vi "read-json-testing.vi"() -> ()   [LabVIEW 2019]
panel:
  out "value":T1(array[cluster])
  in  "trajectory":T1(array[cluster])
  in  "enable LabVIEW extensions? (T)":bool=TRUE
  in  "strict validation? (F)":bool
  in  "default null elements? (F)":bool=TRUE
  out "error out":errorcluster
  in  "path":string[](array[string])
  in  "json source":string="[\n    {\n        \"timestamp\": 0,\n        \"x\": 5.982723236083984,\n        \"y\": 3.8337526321411137,\n        \"heading\": -0.02726589531195272,\n        \"velocityX\": 0,\n        \"velocityY\": 9.683808101189284e-35,\n        \"angularVelocity\": 0\n    },\n    {\n        \"timestamp\": 0.03810324695055001,\n        \"x\": 5.98684701120518,\n        \"y\": 3.836695144747058,\n        \"heading\": -0.02635908015583591,\n        \"velocityX\": 0.10822634424167109,\n        \"velocityY\": 0.07722472076364896,\n        \"angularVelocity\": 0.023798894548105808\n    },\n    {\n        \"timestamp\": 0.07620649390110001,\n        \"x\": 5.9951102276307955,\n        \"y\": 3.842555990890375,\n        \"heading\": -0.02450943734161065,\n        \"velocityX\": 0.21686383935573297,\n        \"velocityY\": 0.15381487438388347,\n        \"angularVelocity\": 0.048542918576604074\n    },\n    {\n        \"timestamp\": 0.11430974085165002,\n        \"x\": 6.007530540708913,\n        \"y\": 3.851307449548468,\n        \"heading\": -0.021675911820365212,\n        \"velocityX\": 0.3259646899445822,\n        \"velocityY\": 0.2296775041100852,\n        \"angularVelocity\": 0.07436441112018764\n    },\n    {\n        \"timestamp\": 0.15241298780220003,\n        \"x\": 6.024127990876516,\n        \"y\": 3.8629174242827835,\n        \"heading\": -0.017811264169326626,\n        \"velocityX\": 0.43559149143231607,\n        \"velocityY\": 0.3046977794145049,\n        \"angularVelocity\": 0.10142567787079011\n    },\n    {\n        \"timestamp\": 0.19051623475275004,\n        \"x\": 6.044925508435204,\n        \"y\": 3.8773483282979404,\n        \"heading\": -0.0128605531052204,\n        \"velocityX\": 0.5458200868203993,\n        \"velocityY\": 0.37873160872313927,\n        \"angularVelocity\": 0.12992885017200875\n    },\n    {\n        \"timestamp\": 0.22861948170330004,\n        \"x\": 6.0699495650843565,\n        \"y\": 3.894555559389049,\n        \"heading\": -0.006759072154586934,\n        \"velocityX\": 0.6567434182611646,\n        \"velocityY\": 0.45159487624347117,\n        \"angularVelocity\": 0.16013021038733294\n    },\n    {\n        \"timestamp\": 0.26672272865385005,\n        \"x\": 6.0992310251847055,\n        \"y\": 3.91448535931083,\n        \"heading\": 0.0005705329934009674,\n        \"velocityX\": 0.7684767688787957,\n        \"velocityY\": 0.5230472864332357,\n        \"angularVelocity\": 0.19236169446395399\n    },\n    {\n        \"timestamp\": 0.30482597560440006,\n        \"x\": 6.132806269868785,\n        \"y\": 3.9370717165814155,\n        \"heading\": 0.009222426006961602,\n        \"velocityX\": 0.8811649234946475,\n        \"velocityY\": 0.5927672594384606,\n        \"angularVelocity\": 0.2270644552887354\n    },\n    {\n        \"timestamp\": 0.34292922255495006,\n        \"x\": 6.170718689966367,\n        \"y\": 3.962231721071589,\n        \"heading\": 0.01931383560441445,\n        \"velocityX\": 0.9949918479857032,\n        \"velocityY\": 0.6603112990035996,\n        \"angularVelocity\": 0.2648438231667591\n    },\n    {\n        \"timestamp\": 0.38103246950550007,\n        \"x\": 6.213020653091169,\n        \"y\": 3.989858289069104,\n        \"heading\": 0.030994951202651673,\n        \"velocityX\": 1.1101931334015223,\n        \"velocityY\": 0.7250449819504136,\n        \"angularVelocity\": 0.3065648345768179\n    },\n    {\n        \"timestamp\": 0.4191357164560501,\n        \"x\": 6.259775973212591,\n        \"y\": 4.019808160211835,\n        \"heading\": 0.04446563724227389,\n        \"velocityX\": 1.2270691834242344,\n        \"velocityY\": 0.7860188708221707,\n        \"angularVelocity\": 0.3535311848122014\n    },\n    {\n        \"timestamp\": 0.4572389634066001,\n        \"x\": 6.311062435579481,\n        \"y\": 4.051880814371457,\n        \"heading\": 0.060006160684953305,\n        \"velocityX\": 1.3459866670536105,\n        \"velocityY\": 0.8417302126835429,\n        \"angularVelocity\": 0.40785299643479905\n    },\n    {\n        \"timestamp\": 0.4953422103571501,\n        \"x\": 6.366971668412108,\n        \"y\": 4.085778739706103,\n        \"heading\": 0.0780398678585479,\n        \"velocityX\": 1.4673088859116663,\n        \"velocityY\": 0.8896335102002109,\n        \"angularVelocity\": 0.47328531337489643\n    },\n    {\n        \"timestamp\": 0.5334454573077001,\n        \"x\": 6.42759324409593,\n        \"y\": 4.1210284288786045,\n        \"heading\": 0.09927318993914273,\n        \"velocityX\": 1.5909818856775562,\n        \"velocityY\": 0.9251098526654346,\n        \"angularVelocity\": 0.5572575509942492\n    },\n    {\n        \"timestamp\": 0.5715487042582501,\n        \"x\": 6.492929850638083,\n        \"y\": 4.156837507973627,\n        \"heading\": 0.12496268004834134,\n        \"velocityX\": 1.7147254307998017,\n        \"velocityY\": 0.9397907517301461,\n        \"angularVelocity\": 0.6742073750968268\n    },\n    {\n        \"timestamp\": 0.6096519512088001,\n        \"x\": 6.562698684949471,\n        \"y\": 4.191947985905663,\n        \"heading\": 0.1565497680971661,\n        \"velocityX\": 1.8310469551829356,\n        \"velocityY\": 0.9214563256930572,\n        \"angularVelocity\": 0.8289867813578368\n    },\n    {\n        \"timestamp\": 0.6477551981593501,\n        \"x\": 6.635139463079909,\n        \"y\": 4.223639351259096,\n        \"heading\": 0.19449877991768647,\n        \"velocityX\": 1.9011707381381133,\n        \"velocityY\": 0.8317234852599791,\n        \"angularVelocity\": 0.9959521788203487\n    },\n    {\n        \"timestamp\": 0.6858584451099001,\n        \"x\": 6.7081933797465005,\n        \"y\": 4.250935758839449,\n        \"heading\": 0.23877166971400077,\n        \"velocityX\": 1.917262241755836,\n        \"velocityY\": 0.7163800926409031,\n        \"angularVelocity\": 1.1619190840553386\n    },\n    {\n        \"timestamp\": 0.7239616920604501,\n        \"x\": 6.780136139474193,\n        \"y\": 4.273495418390116,\n        \"heading\": 0.28647328812510897,\n        \"velocityX\": 1.888100502853595,\n        \"velocityY\": 0.5920665915937995,\n        \"angularVelocity\": 1.2519042923826915\n    },\n    {\n        \"timestamp\": 0.7620649390110001,\n        \"x\": 6.850045632550813,\n        \"y\": 4.291512251071874,\n        \"heading\": 0.3365456853758495,\n        \"velocityX\": 1.8347384716936121,\n        \"velocityY\": 0.47284245106833517,\n        \"angularVelocity\": 1.3141241562884853\n    },\n    {\n        \"timestamp\": 0.8001681859615501,\n        \"x\": 6.9174385893155375,\n        \"y\": 4.305183550968592,\n        \"heading\": 0.3884190669725829,\n        \"velocityX\": 1.7686932783493219,\n        \"velocityY\": 0.35879619168575444,\n        \"angularVelocity\": 1.3613900585442669\n    },\n    {\n        \"timestamp\": 0.8382714329121002,\n        \"x\": 6.982024412284714,\n        \"y\": 4.314663617385671,\n        \"heading\": 0.44170912410253604,\n        \"velocityX\": 1.6950215044138437,\n        \"velocityY\": 0.24879943773254676,\n        \"angularVelocity\": 1.398569974866313\n    },\n    {\n        \"timestamp\": 0.8763746798626502,\n        \"x\": 7.043611527543253,\n        \"y\": 4.320071315528175,\n        \"heading\": 0.49614021122658447,\n        \"velocityX\": 1.616321972205263,\n        \"velocityY\": 0.14192223958037933,\n        \"angularVelocity\": 1.4285157166445919\n    },\n    {\n        \"timestamp\": 0.9144779268132002,\n        \"x\": 7.102065214635615,\n        \"y\": 4.32149953061112,\n        \"heading\": 0.5515071646371278,\n        \"velocityX\": 1.5340867713510038,\n        \"velocityY\": 0.037482765833582746,\n        \"angularVelocity\": 1.4530770430772049\n    },\n    {\n        \"timestamp\": 0.9525811737637502,\n        \"x\": 7.157286057818237,\n        \"y\": 4.319022257662232,\n        \"heading\": 0.6076525295540515,\n        \"velocityX\": 1.4492424557488948,\n        \"velocityY\": -0.06501474669864526,\n        \"angularVelocity\": 1.4735060502794106\n    },\n    {\n        \"timestamp\": 0.9906844207143002,\n        \"x\": 7.209197910760983,\n        \"y\": 4.312699565476428,\n        \"heading\": 0.664452255224938,\n        \"velocityX\": 1.362399719113554,\n        \"velocityY\": -0.1659357847904016,\n        \"angularVelocity\": 1.4906794096734857\n    },\n    {\n        \"timestamp\": 1.0287876676648502,\n        \"x\": 7.2577407022992615,\n        \"y\": 4.302581057423054,\n        \"heading\": 0.7218063948940598,\n        \"velocityX\": 1.2739804458469486,\n        \"velocityY\": -0.2655550081205459,\n        \"angularVelocity\": 1.5052297181801246\n    },\n    {\n        \"timestamp\": 1.0668909146154002,\n        \"x\": 7.3028658963835795,\n        \"y\": 4.288708316667104,\n        \"heading\": 0.779632866785423,\n        \"velocityX\": 1.184287369075913,\n        \"velocityY\": -0.3640829028022947,\n        \"angularVelocity\": 1.51762583294836\n    },\n    {\n        \"timestamp\": 1.1049941615659502,\n        \"x\": 7.344533497015384,\n        \"y\": 4.271116666027759,\n        \"heading\": 0.8378631451292572,\n        \"velocityX\": 1.0935446180184787,\n        \"velocityY\": -0.4616837683721217,\n        \"angularVelocity\": 1.5282235243470785\n    },\n    {\n        \"timestamp\": 1.1430974085165002,\n        \"x\": 7.3827099980564315,\n        \"y\": 4.249836459267662,\n        \"heading\": 0.8964392046934532,\n        \"velocityX\": 1.0019225157003373,\n        \"velocityY\": -0.5584880151477051,\n        \"angularVelocity\": 1.537298373553775\n    },\n    {\n        \"timestamp\": 1.1812006554670502,\n        \"x\": 7.417366935383198,\n        \"y\": 4.22489404631923,\n        \"heading\": 0.9553113025588683,\n        \"velocityX\": 0.9095533871888511,\n        \"velocityY\": -0.6546007215816033,\n        \"angularVelocity\": 1.5450677455866486\n    },\n    {\n        \"timestamp\": 1.2193039024176002,\n        \"x\": 7.448479836830729,\n        \"y\": 4.1963125073290035,\n        \"heading\": 1.014436333735295,\n        \"velocityX\": 0.816541999371032,\n        \"velocityY\": -0.7501077015120999,\n        \"angularVelocity\": 1.551705849455849\n    },\n    {\n        \"timestamp\": 1.2574071493681502,\n        \"x\": 7.4760274429392135,\n        \"y\": 4.164112219770215,\n        \"heading\": 1.0737765893932227,\n        \"velocityX\": 0.7229726680310206,\n        \"velocityY\": -0.8450798852018467,\n        \"angularVelocity\": 1.5573543046066753\n    },\n    {\n        \"timestamp\": 1.2955103963187002,\n        \"x\": 7.49999111698165,\n        \"y\": 4.12831130292246,\n        \"heading\": 1.1332988035654967,\n        \"velocityX\": 0.628914225434282,\n        \"velocityY\": -0.9395765377742389,\n        \"angularVelocity\": 1.5621297116627306\n    },\n    {\n        \"timestamp\": 1.3336136432692502,\n        \"x\": 7.520354390382808,\n        \"y\": 4.08892597080947,\n        \"heading\": 1.1929734104345324,\n        \"velocityX\": 0.5344235736021341,\n        \"velocityY\": -1.0336476616835946,\n        \"angularVelocity\": 1.566129179134875\n    },\n    {\n        \"timestamp\": 1.3717168902198003,\n        \"x\": 7.537102606975847,\n        \"y\": 4.045970815789375,\n        \"heading\": 1.252773957923772,\n        \"velocityX\": 0.43954827825499565,\n        \"velocityY\": -1.1273358167045713,\n        \"angularVelocity\": 1.5694344255451789\n    },\n    {\n        \"timestamp\": 1.4098201371703503,\n        \"x\": 7.550222640729637,\n        \"y\": 3.999459038895289,\n        \"heading\": 1.312676639030204,\n        \"velocityX\": 0.3443284970127743,\n        \"velocityY\": -1.2206775174422342,\n        \"angularVelocity\": 1.5721148694801685\n    },\n    {\n        \"timestamp\": 1.4479233841209003,\n        \"x\": 7.5597026689810605,\n        \"y\": 3.9494026387764034,\n        \"heading\": 1.3726599130276154,\n        \"velocityX\": 0.24879843609460844,\n        \"velocityY\": -1.313704319840455,\n        \"angularVelocity\": 1.574229988201789\n    },\n    {\n        \"timestamp\": 1.4860266310714503,\n        \"x\": 7.56553198821413,\n        \"y\": 3.8958125680834574,\n        \"heading\": 1.4327041960899756,\n        \"velocityX\": 0.15298746693777887,\n        \"velocityY\": -1.4064436755874,\n        \"angularVelocity\": 1.5758311395427256\n    },\n    {\n        \"timestamp\": 1.5241298780220003,\n        \"x\": 7.5677008628845215,\n        \"y\": 3.8386988639831543,\n        \"heading\": 1.492791606127603,\n        \"velocityX\": 0.05692099345774061,\n        \"velocityY\": -1.4989196110878606,\n        \"angularVelocity\": 1.576962984692913\n    },\n    {\n        \"timestamp\": 1.564961546846248,\n        \"x\": 7.573888102497922,\n        \"y\": 3.7818679617757693,\n        \"heading\": 1.5572134986128423,\n        \"velocityX\": 0.15153041233834258,\n        \"velocityY\": -1.3918339329211034,\n        \"angularVelocity\": 1.5777433139589185\n    },\n    {\n        \"timestamp\": 1.605793215670496,\n        \"x\": 7.583928738356132,\n        \"y\": 3.7294180830284507,\n        \"heading\": 1.6216492084044356,\n        \"velocityX\": 0.24590314692813534,\n        \"velocityY\": -1.2845391887625002,\n        \"angularVelocity\": 1.5780817107659115\n    },\n    {\n        \"timestamp\": 1.6466248844947438,\n        \"x\": 7.597812163368718,\n        \"y\": 3.681358537835685,\n        \"heading\": 1.6860789847473923,\n        \"velocityX\": 0.34001610544853655,\n        \"velocityY\": -1.177016432995396,\n        \"angularVelocity\": 1.5779363958961614\n    },\n    {\n        \"timestamp\": 1.6874565533189916,\n        \"x\": 7.615526682956808,\n        \"y\": 3.637699519534437,\n        \"heading\": 1.7504811177254895,\n        \"velocityX\": 0.4338426544440016,\n        \"velocityY\": -1.069244034309975,\n        \"angularVelocity\": 1.5772593879350625\n    },\n    {\n        \"timestamp\": 1.7282882221432394,\n        \"x\": 7.637059339376509,\n        \"y\": 3.5984522360053632,\n        \"heading\": 1.8148316323025202,\n        \"velocityX\": 0.5273518579998424,\n        \"velocityY\": -0.9611971457254432,\n        \"angularVelocity\": 1.5759952122950966\n    },\n    {\n        \"timestamp\": 1.7691198909674872,\n        \"x\": 7.662395696195494,\n        \"y\": 3.5636290681903535,\n        \"heading\": 1.8791039149175528,\n        \"velocityX\": 0.6205075018618541,\n        \"velocityY\": -0.8528470380404654,\n        \"angularVelocity\": 1.574079249410144\n    },\n    {\n        \"timestamp\": 1.809951559791735,\n        \"x\": 7.691519570992391,\n        \"y\": 3.5332437632048217,\n        \"heading\": 1.9432682526933631,\n        \"velocityX\": 0.7132668253716068,\n        \"velocityY\": -0.7441602525804,\n        \"angularVelocity\": 1.5714355945625587\n    },\n    {\n        \"timestamp\": 1.8507832286159829,\n        \"x\": 7.72441269980617,\n        \"y\": 3.507311671935531,\n        \"heading\": 2.007291257898031,\n        \"velocityX\": 0.805578849969649,\n        \"velocityY\": -0.6350975117110675,\n        \"angularVelocity\": 1.567974247642089\n    },\n    {\n        \"timestamp\": 1.8916148974402307,\n        \"x\": 7.761054310174422,\n        \"y\": 3.4858500445720093,\n        \"heading\": 2.0711351395192956,\n        \"velocityX\": 0.8973821404647174,\n        \"velocityY\": -0.5256122999992441,\n        \"angularVelocity\": 1.563587368815906\n    },\n    {\n        \"timestamp\": 1.9324465662644785,\n        \"x\": 7.8014205695289,\n        \"y\": 3.4688784026403385,\n        \"heading\": 2.1347567677887986,\n        \"velocityX\": 0.9886017524345373,\n        \"velocityY\": -0.4156489906087677,\n        \"angularVelocity\": 1.5581442077068588\n    },\n    {\n        \"timestamp\": 1.9732782350887264,\n        \"x\": 7.845483860168917,\n        \"y\": 3.4564190136113133,\n        \"heading\": 2.1981064530629975,\n        \"velocityX\": 1.0791449849791273,\n        \"velocityY\": -0.30514033317260225,\n        \"angularVelocity\": 1.5514841077615236\n    },\n    {\n        \"timestamp\": 2.014109903912974,\n        \"x\": 7.893211807339716,\n        \"y\": 3.448497505357414,\n        \"heading\": 2.261126322126411,\n        \"velocityX\": 1.168895334066148,\n        \"velocityY\": -0.19400402878448852,\n        \"angularVelocity\": 1.5434066468033365\n    },\n    {\n        \"timestamp\": 2.054941572737222,\n        \"x\": 7.944565946441019,\n        \"y\": 3.445143674787076,\n        \"heading\": 2.3237481128062893,\n        \"velocityX\": 1.2577036545419125,\n        \"velocityY\": -0.08213797444264499,\n        \"angularVelocity\": 1.533657391017405\n    },\n    {\n        \"timestamp\": 2.09577324156147,\n        \"x\": 7.999499846458567,\n        \"y\": 3.4463925714516828,\n        \"heading\": 2.3858901030926365,\n        \"velocityX\": 1.3453748426007262,\n        \"velocityY\": 0.03058647125063885,\n        \"angularVelocity\": 1.5219066982990461\n    },\n    {\n        \"timestamp\": 2.1366049103857176,\n        \"x\": 8.057956384260022,\n        \"y\": 3.452285978695619,\n        \"heading\": 2.447452706752575,\n        \"velocityX\": 1.4316470397785264,\n        \"velocityY\": 0.1443342242342635,\n        \"angularVelocity\": 1.5077170596413056\n    },\n    {\n        \"timestamp\": 2.1774365792099655,\n        \"x\": 8.11986363569219,\n        \"y\": 3.462874481468067,\n        \"heading\": 2.508311925925005,\n        \"velocityX\": 1.5161577573190377,\n        \"velocityY\": 0.2593208428003823,\n        \"angularVelocity\": 1.4904906148801191\n    },\n    {\n        \"timestamp\": 2.2182682480342133,\n        \"x\": 8.185128396146618,\n        \"y\": 3.4782204145569087,\n        \"heading\": 2.5683091763759016,\n        \"velocityX\": 1.598385819970941,\n        \"velocityY\": 0.3758340898310503,\n        \"angularVelocity\": 1.469380316272348\n    },\n    {\n        \"timestamp\": 2.259099916858461,\n        \"x\": 8.253625378823767,\n        \"y\": 3.498402135996597,\n        \"heading\": 2.627234557026799,\n        \"velocityX\": 1.677545509393189,\n        \"velocityY\": 0.4942663873612369,\n        \"angularVelocity\": 1.4431293735393322\n    },\n    {\n        \"timestamp\": 2.299931585682709,\n        \"x\": 8.325177903992097,\n        \"y\": 3.5235202051846817,\n        \"heading\": 2.6847972126928403,\n        \"velocityX\": 1.7523781718624016,\n        \"velocityY\": 0.6151614644065581,\n        \"angularVelocity\": 1.4097551563178585\n    },\n    {\n        \"timestamp\": 2.3407632545069568,\n        \"x\": 8.399520165830122,\n        \"y\": 3.5537056177972803,\n        \"heading\": 2.7405671841117947,\n        \"velocityX\": 1.820701038647485,\n        \"velocityY\": 0.7392647296031375,\n        \"angularVelocity\": 1.365850895269809\n    },\n    {\n        \"timestamp\": 2.3815949233312046,\n        \"x\": 8.476214939455824,\n        \"y\": 3.5891254614190196,\n        \"heading\": 2.7938439408795164,\n        \"velocityX\": 1.878315920806788,\n        \"velocityY\": 0.8674601024562811,\n        \"angularVelocity\": 1.3047900882289871\n    },\n    {\n        \"timestamp\": 2.4224265921554524,\n        \"x\": 8.55445641673558,\n        \"y\": 3.629944911690221,\n        \"heading\": 2.843312258894989,\n        \"velocityX\": 1.9161959217616398,\n        \"velocityY\": 0.9997007579314489,\n        \"angularVelocity\": 1.2115183983394033\n    },\n    {\n        \"timestamp\": 2.4632582609797002,\n        \"x\": 8.63270684819373,\n        \"y\": 3.6760250979155664,\n        \"heading\": 2.8865347413407387,\n        \"velocityX\": 1.91641521670224,\n        \"velocityY\": 1.1285403597803692,\n        \"angularVelocity\": 1.058552924491086\n    },\n    {\n        \"timestamp\": 2.504089929803948,\n        \"x\": 8.70731172182322,\n        \"y\": 3.7253996813040025,\n        \"heading\": 2.922276108950885,\n        \"velocityX\": 1.8271326099998109,\n        \"velocityY\": 1.2092227628744916,\n        \"angularVelocity\": 0.8753344803012834\n    },\n    {\n        \"timestamp\": 2.544921598628196,\n        \"x\": 8.777061536831155,\n        \"y\": 3.7753594853432584,\n        \"heading\": 2.949709380191114,\n        \"velocityX\": 1.7082283682345663,\n        \"velocityY\": 1.2235552814236639,\n        \"angularVelocity\": 0.6718626015088779\n    },\n    {\n        \"timestamp\": 2.5857532674524437,\n        \"x\": 8.841475923005714,\n        \"y\": 3.823979349131039,\n        \"heading\": 2.9725228149804273,\n        \"velocityX\": 1.5775594784484608,\n        \"velocityY\": 1.1907390804194327,\n        \"angularVelocity\": 0.5587191375275982\n    },\n    {\n        \"timestamp\": 2.6265849362766915,\n        \"x\": 8.900725127375773,\n        \"y\": 3.870275138965792,\n        \"heading\": 2.9920719682931938,\n        \"velocityX\": 1.451060073618111,\n        \"velocityY\": 1.1338206634173846,\n        \"angularVelocity\": 0.4787742915161657\n    },\n    {\n        \"timestamp\": 2.6674166051009394,\n        \"x\": 8.954991259763695,\n        \"y\": 3.913751195609642,\n        \"heading\": 3.009010373474175,\n        \"velocityX\": 1.3290206829777829,\n        \"velocityY\": 1.0647631580031653,\n        \"angularVelocity\": 0.41483499618584174\n    },\n    {\n        \"timestamp\": 2.708248273925187,\n        \"x\": 9.004413690363393,\n        \"y\": 3.9541157023660385,\n        \"heading\": 3.023743409149255,\n        \"velocityX\": 1.210394579081024,\n        \"velocityY\": 0.9885588299154339,\n        \"angularVelocity\": 0.360823745374801\n    },\n    {\n        \"timestamp\": 2.749079942749435,\n        \"x\": 9.049097789798745,\n        \"y\": 3.9911778957153943,\n        \"heading\": 3.0365503891819805,\n        \"velocityX\": 1.09434908545349,\n        \"velocityY\": 0.9076825517193372,\n        \"angularVelocity\": 0.31365311292665315\n    },\n    {\n        \"timestamp\": 2.789911611573683,\n        \"x\": 9.089124874577477,\n        \"y\": 4.02480391238427,\n        \"heading\": 3.0476356317929376,\n        \"velocityX\": 0.9802950976856478,\n        \"velocityY\": 0.8235278556360364,\n        \"angularVelocity\": 0.2714863959801188\n    },\n    {\n        \"timestamp\": 2.8307432803979307,\n        \"x\": 9.124559199537389,\n        \"y\": 4.054894899911004,\n        \"heading\": 3.0571549364034576,\n        \"velocityX\": 0.8678147619298414,\n        \"velocityY\": 0.7369521842531842,\n        \"angularVelocity\": 0.2331353306054306\n    },\n    {\n        \"timestamp\": 2.8715749492221785,\n        \"x\": 9.15545264765326,\n        \"y\": 4.08137499834509,\n        \"heading\": 3.0652309054795936,\n        \"velocityX\": 0.7566050814344037,\n        \"velocityY\": 0.6485186424307532,\n        \"angularVelocity\": 0.19778689700121527\n    },\n    {\n        \"timestamp\": 2.9124066180464263,\n        \"x\": 9.181847907790585,\n        \"y\": 4.1041842207712955,\n        \"heading\": 3.0719624536763006,\n        \"velocityX\": 0.6464408851605111,\n        \"velocityY\": 0.5586159734097851,\n        \"angularVelocity\": 0.1648609618596868\n    },\n    {\n        \"timestamp\": 2.953238286870674,\n        \"x\": 9.203780676978399,\n        \"y\": 4.123273979904036,\n        \"heading\": 3.077431020092421,\n        \"velocityX\": 0.537150937479908,\n        \"velocityY\": 0.4675233631744787,\n        \"angularVelocity\": 0.13392953493168003\n    },\n    {\n        \"timestamp\": 2.994069955694922,\n        \"x\": 9.221281224251845,\n        \"y\": 4.138604141776491,\n        \"heading\": 3.081704794247388,\n        \"velocityX\": 0.4286023025112106,\n        \"velocityY\": 0.3754478402153836,\n        \"angularVelocity\": 0.10466812349403944\n    },\n    {\n        \"timestamp\": 3.03490162451917,\n        \"x\": 9.23437552715582,\n        \"y\": 4.150141009015649,\n        \"heading\": 3.084841687848118,\n        \"velocityX\": 0.32068987824956363,\n        \"velocityY\": 0.2825470418271738,\n        \"angularVelocity\": 0.07682501575503786\n    },\n    {\n        \"timestamp\": 3.0757332933434176,\n        \"x\": 9.243086115335979,\n        \"y\": 4.157855895393255,\n        \"heading\": 3.0868914836292065,\n        \"velocityX\": 0.2133292229042485,\n        \"velocityY\": 0.18894369492496685,\n        \"angularVelocity\": 0.05020112672616272\n    },\n    {\n        \"timestamp\": 3.1165649621676654,\n        \"x\": 9.247432708740234,\n        \"y\": 4.161724090576172,\n        \"heading\": 3.087897426551899,\n        \"velocityX\": 0.10645152474578339,\n        \"velocityY\": 0.09473517233807482,\n        \"angularVelocity\": 0.024636341145439937\n    },\n    {\n        \"timestamp\": 3.1573966309919133,\n        \"x\": 9.247432708740234,\n        \"y\": 4.161724090576172,\n        \"heading\": 3.087897426551899,\n        \"velocityX\": 7.74756381521956e-33,\n        \"velocityY\": 1.0517742336989922e-32,\n        \"angularVelocity\": 0\n    }\n]"
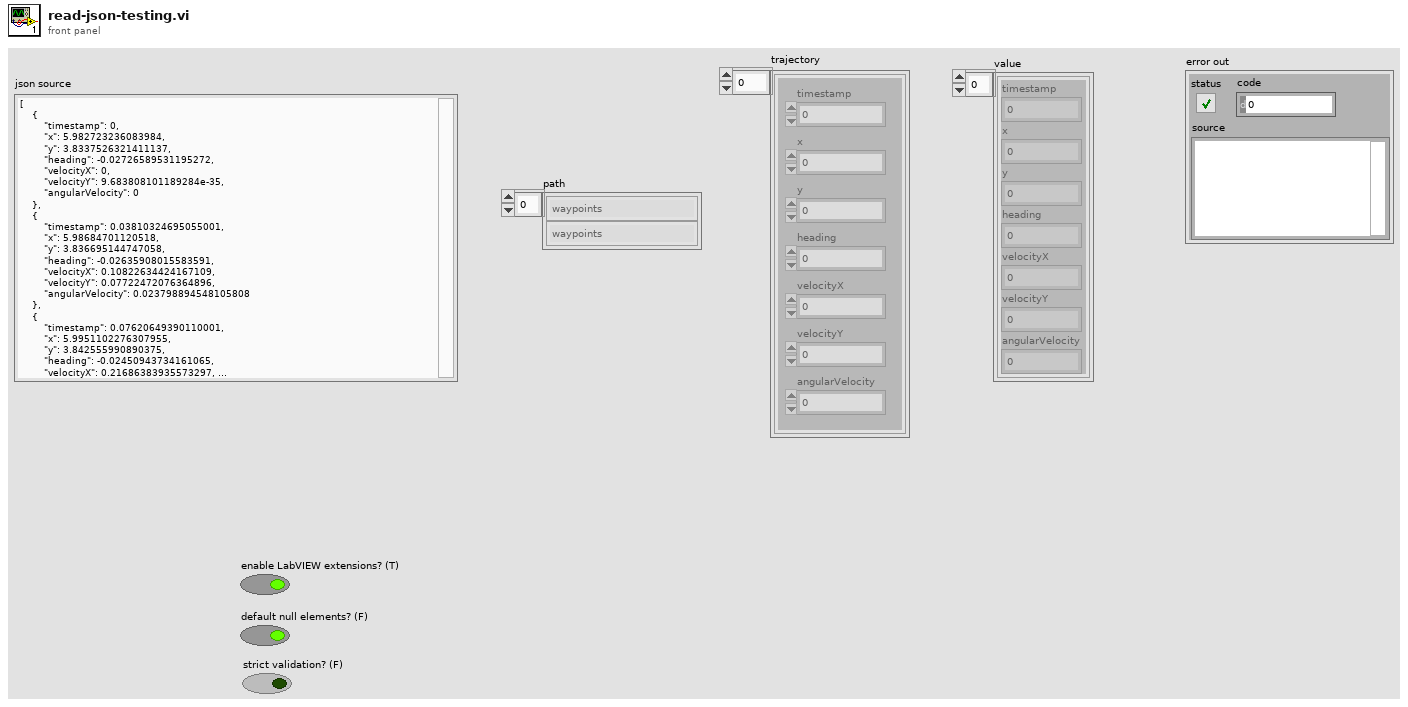
[diagram p1: front panel]
types:
  T1 = cluster{"timestamp":dbl, "x":dbl, "y":dbl, "heading":dbl, "velocityX":dbl, "velocityY":dbl, "angularVelocity":dbl}[]
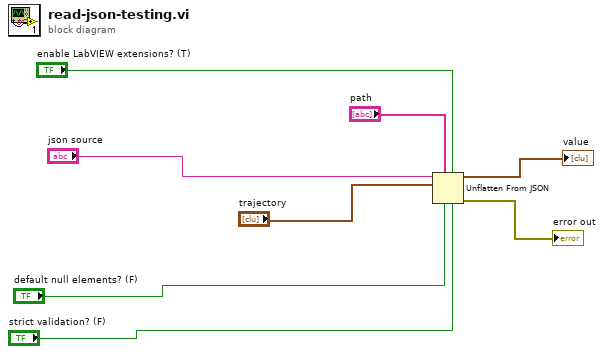
[diagram p0: block diagram]
diagram:
  n1 = Unflatten From JSON(path="path", enable LabVIEW extensions? (T)="enable LabVIEW extensions? (T)", JSON string="json source", type and defaults="trajectory", default null elements? (F)="default null elements? (F)", strict validation? (F)="strict validation? (F)") -> (value=→"value":T1, error out=→"error out":errorcluster)  [unwired: 1 in]
